vi "Game Simon Say.vi"() -> ()   [LabVIEW 2021, in "Scrach.lvlib"]
uses:
  JavierLopez/#32 Simon Says/Scrach.lvlib
  Transporter/Transporter.lvclass
  ShiftR/ShiftR.lvclass
  Class 2/Close.lvclass
  Start/Start.lvclass
  Case A/Case Red.lvclass
  D:/Repository/OOP_SimonSay/Abstract/Abstract.lvclass
  D:/Repository/OOP_SimonSay/Case A/Case Red.lvclass
  Initialize/Initialize.lvclass
  Abstract/Abstract.lvclass
  D:/Repository/OOP_SimonSay/Initialize/Initialize.lvclass
  D:/Repository/OOP_SimonSay/Class 2/Close.lvclass
  D:/Repository/OOP_SimonSay/Start/Start.lvclass
  Control/Purple ButonCtlr.ctl
  Control/Start.ctl
  Control/Red Buton Indicator.ctl
  Control/Green Buton Indicator.ctl
  Control/Orange Buton Indicator.ctl
  Control/Blue Buton Indicator.ctl
panel:
  out "SCORE":string
  in  "3":T1
  in  "Start":T2
  in  "5":T3
  in  "1":T4
  in  "2":T5
  in  "4":T6
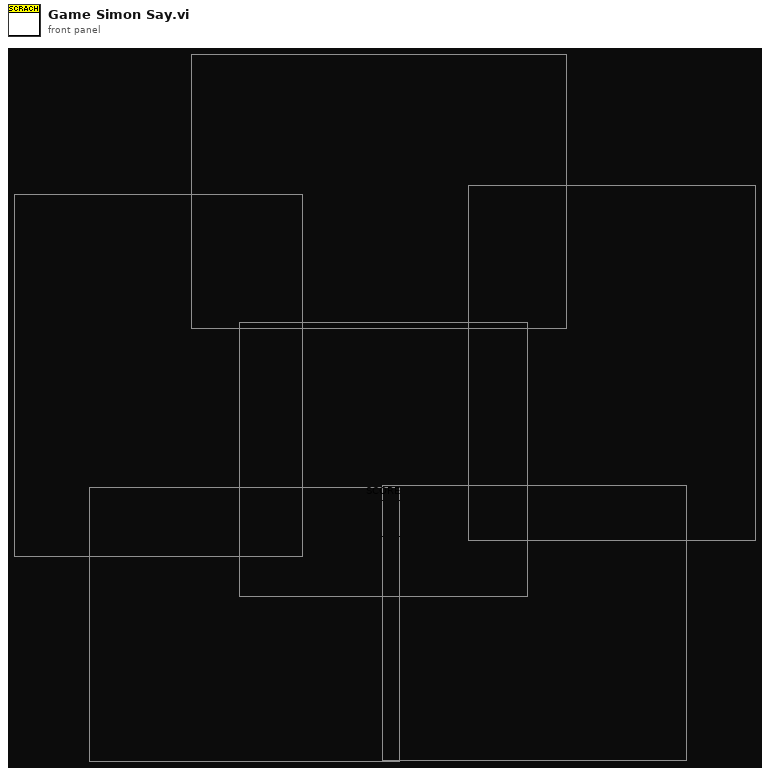
[diagram p1: front panel]
types:
  T1 = typedef "Orange Buton Indicator.ctl" = bool
  T2 = typedef "Start.ctl" = bool
  T3 = typedef "Purple ButonCtlr.ctl" = bool
  T4 = typedef "Red Buton Indicator.ctl" = bool
  T5 = typedef "Green Buton Indicator.ctl" = bool
  T6 = typedef "Blue Buton Indicator.ctl" = bool
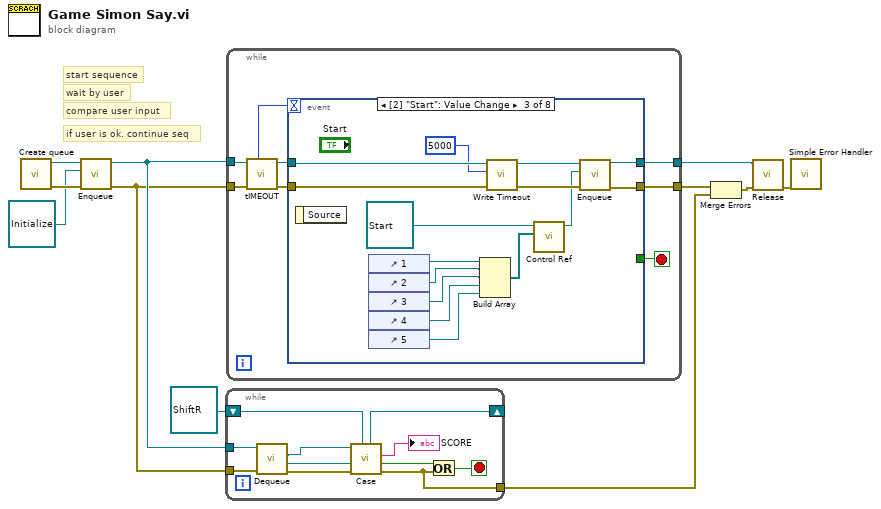
[diagram p0: block diagram]
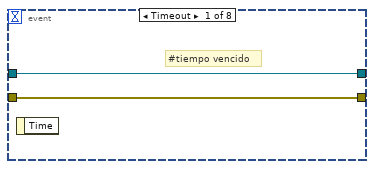
[diagram p2: hidden frame]
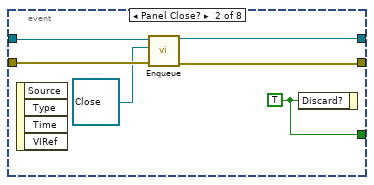
[diagram p3: hidden frame]
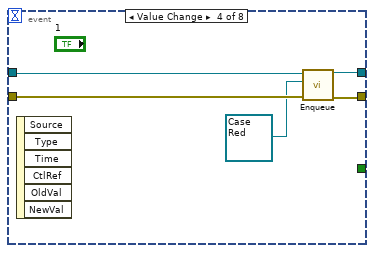
[diagram p4: hidden frame]
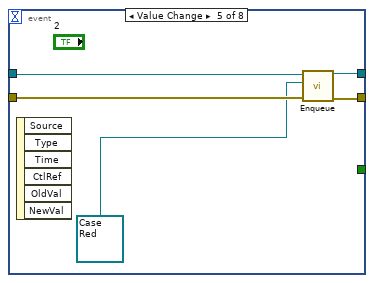
[diagram p5: hidden frame]
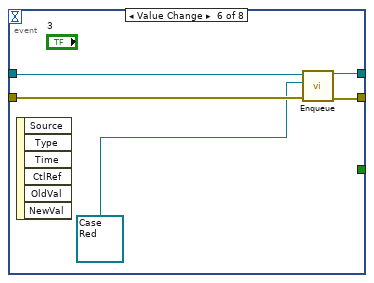
[diagram p6: hidden frame]
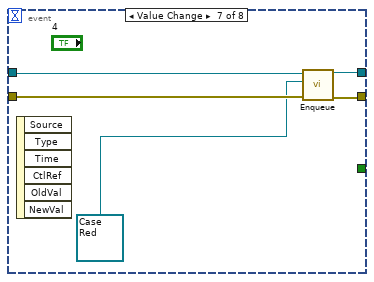
[diagram p7: hidden frame]
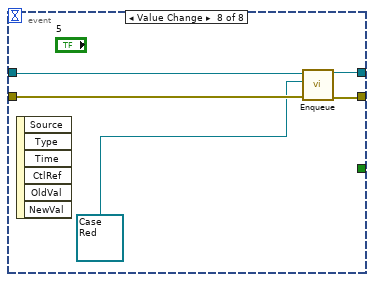
[diagram p8: hidden frame]
diagram:
  # "if user is ok. continue seq"
  # "compare user input"
  # "wait by user"
  # "start sequence"
  n1 = call "Create queue.vi"() -> ("error out"=w5:errorcluster, "Transporter out"=w4:refnum<class "Transporter.lvclass">)  [unwired: 10 in]
  n2 = call-dynamic "Enqueue.vi"("error in (no error)"=w5, "Abstract"=refnum<class "Initialize.lvclass"> refnum ("Msn Trasnsportation Library 1.lvlib:Initialize.lvclass"), "Transporter in"=w4) -> ("error out"=w2:errorcluster, "Transporter out"=w3:refnum<class "Transporter.lvclass">)  [unwired: 7 in]
  n3 = while {
    tunnel: w2 -> [w22]
    tunnel: w3 -> [w14]
    shift-right: [w16] -> _
    shift-left: refnum<class "ShiftR.lvclass"> refnum ("Msn Trasnsportation Library 1.lvlib:ShiftR.lvclass") -> [w17]
    tunnel: [w18] -> w6
    stop <- w19 stop-if-true
    n4 = call "Dequeue.vi"("error in"=w22, "Transporter in"=w14) -> ("error out"=w21:errorcluster, "queue out"=w12:refnum<queue>, "Abstract"=w13:refnum<class "Abstract.lvclass">)  [unwired: 7 in]
    n5 = call-dynamic "Case.vi"("ShiftR"=w17, "error in (no error)"=w21, "queue In"=w12, "Abstract in"=w13) -> ("error out"=w18:errorcluster, "Exit"=w20:bool, "Scrore"=→"SCORE":string, "ShiftR out"=w16:refnum<class "ShiftR.lvclass">)  [unwired: 3 in, 1 out]
    n6 = Or(x=w20, y=w18) -> (x .or. y?=w19:bool)
  }
  n7 = while {
    tunnel: w3 -> [w25]
    tunnel: [w29] -> w11
    tunnel: w2 -> [w28]
    tunnel: [w27] -> w10
    stop <- w26 stop-if-true
    n8 = call-dynamic "tIMEOUT.vi"("Transporter in"=w25) -> ("Transporter out"=w24:refnum<class "Transporter.lvclass">, "Timeout"=w23:i32)  [unwired: 9 in]
    n9 = event shown="[2] \"Start\": Value Change" {
      selector: _ -> [_ _ _ _ _ _ _ _]
      dyn-events: _ -> [_ _ _ _ _ _ _ _]
      timeout: w23 -> [_ _ _ _ _ _ _ _]
      tunnel: [w31 w37 w51 w56 w61 w66 w71 w76] -> w29
      tunnel: w24 -> [w31 w36 w40 w55 w60 w65 w70 w75]
      tunnel: w28 -> [w30 w35 w50 w54 w59 w64 w69 w74]
      tunnel: [w30 w34 w49 w53 w58 w63 w68 w73] -> w27
      tunnel: [_ w32 _ _ _ _ _ _] -> w26
      event Timeout {
        # "#tiempo vencido"
        n10 = event-data() -> ()  [unwired: 1 in, 1 out]
      }
      event Panel Close? {
        w32 = TRUE ("Discard?")
        n11 = event-data() -> ()  [unwired: 1 in, 4 out]
        n12 = call-dynamic "Enqueue.vi"("error in (no error)"=w35, "Abstract"=refnum<class "Close.lvclass"> refnum ("Msn Trasnsportation Library 1.lvlib:Close.lvclass"), "Transporter in"=w36) -> ("error out"=w34:errorcluster, "Transporter out"=w37:refnum<class "Transporter.lvclass">)  [unwired: 7 in]
        n13 = event-data("Discard?"=w32) -> ()  [unwired: 1 in, 1 out]
      }
      event Value Change {
        n14 = event-data() -> ()  [unwired: 1 in, 1 out]
        n15 = control-ref of="1"() -> (w45:refnum<vi>)
        n16 = control-ref of="2"() -> (w44:refnum<vi>)
        n17 = control-ref of="3"() -> (w43:refnum<vi>)
        n18 = control-ref of="4"() -> (w42:refnum<vi>)
        n19 = control-ref of="5"() -> (w41:refnum<vi>)
        n20 = Build Array(w45, w44, w43, w42, w41) -> (w46:refnum<vi>[])
        n21 = call-dynamic "Write Timeout.vi"("Timeout"=5000, "Transporter in"=w40) -> ("Transporter out"=w39:refnum<class "Transporter.lvclass">)  [unwired: 9 in]
        n22 = call-dynamic "Control Ref.vi"("Ctl"=w46, "Start in"=refnum<class "Start.lvclass"> refnum ("Msn Trasnsportation Library 1.lvlib:Start.lvclass")) -> ("Start out"=w47:refnum<class "Start.lvclass">)  [unwired: 8 in, 1 out]
        n23 = call-dynamic "Enqueue.vi"("error in (no error)"=w50, "Abstract"=w47, "Transporter in"=w39) -> ("error out"=w49:errorcluster, "Transporter out"=w51:refnum<class "Transporter.lvclass">)  [unwired: 7 in]
      }
      event Value Change {
        n24 = event-data() -> ()  [unwired: 1 in, 6 out]
        n25 = call-dynamic "Enqueue.vi"("error in (no error)"=w54, "Abstract"=refnum<class "Case Red.lvclass"> refnum ("Msn Trasnsportation Library 1.lvlib:Case A.lvclass"), "Transporter in"=w55) -> ("error out"=w53:errorcluster, "Transporter out"=w56:refnum<class "Transporter.lvclass">)  [unwired: 7 in]
      }
      event Value Change {
        n26 = event-data() -> ()  [unwired: 1 in, 6 out]
        n27 = call-dynamic "Enqueue.vi"("error in (no error)"=w59, "Abstract"=refnum<class "Case Red.lvclass"> refnum ("Msn Trasnsportation Library 1.lvlib:Case A.lvclass"), "Transporter in"=w60) -> ("error out"=w58:errorcluster, "Transporter out"=w61:refnum<class "Transporter.lvclass">)  [unwired: 7 in]
      }
      event Value Change {
        n28 = event-data() -> ()  [unwired: 1 in, 6 out]
        n29 = call-dynamic "Enqueue.vi"("error in (no error)"=w64, "Abstract"=refnum<class "Case Red.lvclass"> refnum ("Msn Trasnsportation Library 1.lvlib:Case A.lvclass"), "Transporter in"=w65) -> ("error out"=w63:errorcluster, "Transporter out"=w66:refnum<class "Transporter.lvclass">)  [unwired: 7 in]
      }
      event Value Change {
        n30 = event-data() -> ()  [unwired: 1 in, 6 out]
        n31 = call-dynamic "Enqueue.vi"("error in (no error)"=w69, "Abstract"=refnum<class "Case Red.lvclass"> refnum ("Msn Trasnsportation Library 1.lvlib:Case A.lvclass"), "Transporter in"=w70) -> ("error out"=w68:errorcluster, "Transporter out"=w71:refnum<class "Transporter.lvclass">)  [unwired: 7 in]
      }
      event Value Change {
        n32 = event-data() -> ()  [unwired: 1 in, 6 out]
        n33 = call-dynamic "Enqueue.vi"("error in (no error)"=w74, "Abstract"=refnum<class "Case Red.lvclass"> refnum ("Msn Trasnsportation Library 1.lvlib:Case A.lvclass"), "Transporter in"=w75) -> ("error out"=w73:errorcluster, "Transporter out"=w76:refnum<class "Transporter.lvclass">)  [unwired: 7 in]
      }
    }
  }
  n34 = Merge Errors(w10, w6) -> (w7:errorcluster)
  n35 = call-dynamic "Release.vi"("error in (no error)"=w7, "Transporter in"=w11) -> ("error out"=w9:errorcluster)  [unwired: 9 in]
  n36 = call <vilib>:"Simple Error Handler.vi"("error in (no error)"=w9) -> ()  [unwired: 4 in, 5 out]
